vi "OnValueChange_leftUserOne.vi"(8 "error in (no error)":errorcluster, 9 "Value":bool, 11 "Game in":refnum<class "Game.lvclass">) -> (0 "error out":errorcluster, 3 "Game out":refnum<class "Game.lvclass">)   [LabVIEW 2019, in "RT_Game.lvlib" / "Game.lvclass"]
uses:
  Game.lvclass
  Engine/ChangeVolumeData.ctl
  Engine/Engine.lvclass
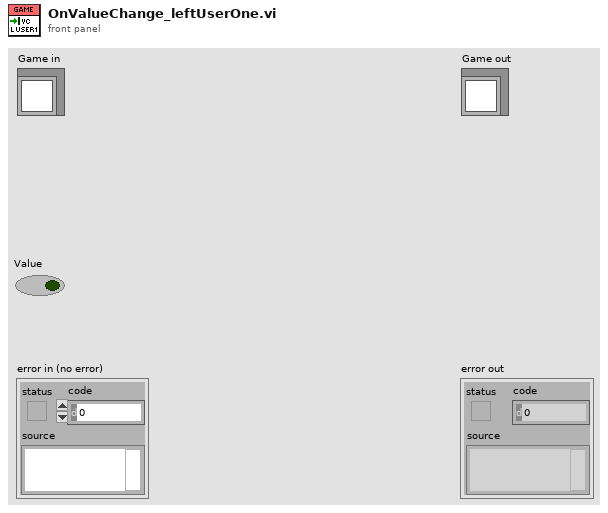
[diagram p1: front panel]
types:
  T1 = typedef "RT_Game.lvlib/Engine.lvclass/ChangeVolumeData.ctl" = enum16{"up", "down", "mute"}
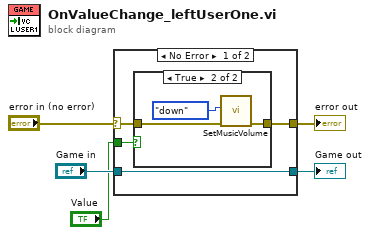
[diagram p0: block diagram]
diagram:
  n1 = case shown="No Error" "error in (no error)" {
    selector: "error in (no error)" -> [w8 w15]
    tunnel: [w7 w15] -> w4
    tunnel: [w9 w14] -> w2
    tunnel: "Game in" -> [w9 w14]
    tunnel: "Value" -> [w6 _]
    frame No Error {
      n2 = case shown="True" w6 {
        tunnel: w8 -> [w10 w13]
        tunnel: [w10 w12] -> w7
        frame False {
        }
        frame True {
          n3 = call "SetMusicVolume.vi"("error in (no error)"=w13, "VolumeData"=ChangeVolumeData."down") -> ("error out"=w12:errorcluster)  [unwired: 9 in]
        }
      }
    }
    frame Error {
    }
  }
  "error out" <- w4
  "Game out" <- w2
